vi "FastCalib.vi"(0 "Pixel to micron":dbl=1.58, 1 "No of each images":dbl, 2 "Template Path":path, 3 "coordinates":dbl[][](array[numeric]), 4 "Array 2":T2[](array[plugin-control])) -> (7 "angle in radian.":dbl, 8 "Mean":dbl[][](array[numeric]))   [LabVIEW 2016]
uses:
  <vilib>/vision/Measure.llb/Edge Options.ctl
  <vilib>/vision/Measure.llb/Edge Polarity.ctl
  <vilib>/Analysis/6fits.llb/Curve Fitting Criteria.ctl
  <vilib>/vision/NI_Vision_Development_Module.lvlib
  <resource>/objmgr/IMAQImage.rc
  <vilib>/Analysis/NI_AALBase.lvlib
  <vilib>/Analysis/NI_AALPro.lvlib
panel:
  in  "Tab Control":T1(tab)
  out "Y pixel":dbl
  out "X pixel":dbl
  out "angle.":dbl
  out "standard deviation":dbl[][](array[numeric])
  out "ratio of good position.":dbl[](array[numeric])
  in  "method":T3 items=["Least Square", "Least Absolute Residual", "Bisquare"]
  in  "Settings":T4={"Algorithm"=1, "Number of Matches Requested"=1, "Minimum Match Score"=800.0, "SubPixel Accuracy"=TRUE, "Rotation Angle Ranges"=[{"Start"=0.0, "End"=360.0}], "Show Search Area"=FALSE, "Show Result"=TRUE} {"Rotation Angle Ranges"."End" format="%.1f"; "Rotation Angle Ranges"."Start" format="%.1f"; "Minimum Match Score" min=0 max=1000 format="%.2f"; "Number of Matches Requested" min=1; "Algorithm" items=["All", "Low Discrepancy Sampling", "Grayscale Value Pyramid", "Gradients Pyramid"]}
  in  "Circle Fit Options":T5={"Process"=enum."Get First Edge", "Step Size"=3.0, "Max Pixel Radius"=3}
  in  "Options":T8={"Search  Direction"=1, "Edge Options"={"Edge Polarity"=0, "Kernel Size"=3, "Width"=3, "Minimum Edge Strength"=10.0, "Interpolation Type"=enum."Bilinear Fixed", "Data Processing Method"=enum."Average"}, "Show Search Area"=FALSE, "Show Search Lines"=FALSE, "Show Edges Found"=FALSE, "Show Result"=TRUE, "Search Area Color"=65280, "Search Lines Color"=255, "Edge Locations Color"=16776960, "Result Color"=16711680, "Overlay Group Name"=""} {"Search  Direction" items=["Outside to Inside", "Inside to Outside"]; "Edge Options"."Edge Polarity" items=["All Edges", "Rising Edges", "Falling Edges"]; "Edge Options"."Minimum Edge Strength" format="%.2f"; "Edge Options"."Width" step=2; "Edge Options"."Kernel Size" step=2}
  in  "Annulus ROI Descriptor":T9={"Global Rectangle"=[675, 567, 1751, 1642], "Contours"=[{"ID"=enum."External", "Type"=7, "Coordinates"=[1212, 1104, 85, 537, 0, 0]}]} {"Contours"."Type" items=["No Selection", "Point", "Line", "Rectangle", "Oval", "Polygon", "Freehand Region", "Annulus", "Unused2", "Unused3", "Broken Line", "Freehand Line", "Rotated Rectangle"]}
  out "Fitted Circle":T10 {"Average SNR (dB)" format="%.2f"; "Average Strength" format="%.2f"; "Roundness (Real-World)" format="%.2f"; "Radius (Real-World)" format="%.2f"; "Center (Real-World)"."Y" format="%.2f"; "Center (Real-World)"."X" format="%.2f"; "Radius (Pixels)" format="%.2f"; "Center (Pixels)"."Y" format="%.2f"; "Center (Pixels)"."X" format="%.2f"}
  out "Resulting ROI":T11
  out "Array":T2[](array[plugin-control])
  in  "No of pin":dbl=7.0
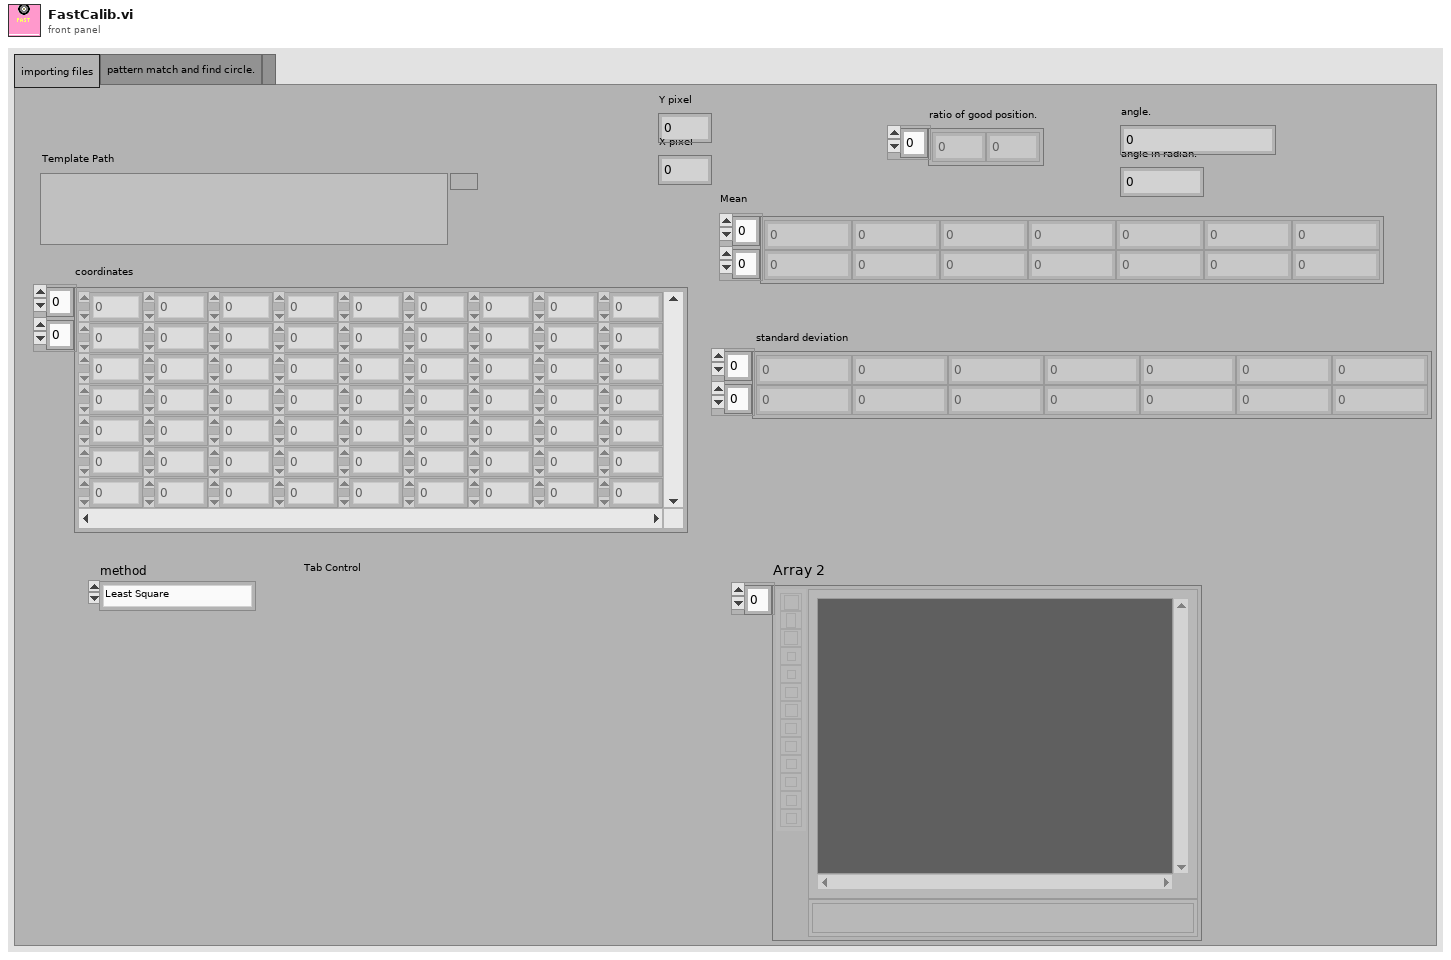
[diagram p1: front panel]
types:
  T1 = enum32{"importing files", "pattern match and find circle.", ""}
  T2 = typedef "IMAQ Image.ctl" = refnum<image>
  T3 = typedef "NI_AALPro.lvlib/Curve Fitting Criteria.ctl" = u16
  T4 = cluster{"Algorithm":i32, "Number of Matches Requested":i32, "Minimum Match Score":sgl, "SubPixel Accuracy":bool, "Rotation Angle Ranges":cluster{"Start":sgl, "End":sgl}[], "Show Search Area":bool, "Show Result":bool}
  T5 = cluster{"Process":enum16{"Get First Edge", "Get First + Last Edge", "Get All Edges", "Get Best Edge"}, "Step Size":dbl, "Max Pixel Radius":i32}
  T6 = typedef "Edge Options.ctl" = cluster{"Edge Polarity":T7, "Kernel Size":u32, "Width":u32, "Minimum Edge Strength":sgl, "Interpolation Type":enum32{"Zero Order", "Bilinear", "Quadratic", "Cubic", "Bilinear Fixed"}, "Data Processing Method":enum32{"Average", "Median"}}
  T7 = typedef "Edge Polarity.ctl" = u32
  T8 = cluster{"Search  Direction":u32, "Edge Options":T6, "Show Search Area":bool, "Show Search Lines":bool, "Show Edges Found":bool, "Show Result":bool, "Search Area Color":u32, "Search Lines Color":u32, "Edge Locations Color":u32, "Result Color":u32, "Overlay Group Name":string}
  T9 = cluster{"Global Rectangle":i32[], "Contours":cluster{"ID":enum32{"External", "Internal"}, "Type":u32, "Coordinates":i32[]}[]}
  T10 = cluster{"Center (Pixels)":cluster{"X":sgl, "Y":sgl}, "Radius (Pixels)":dbl, "Center (Real-World)":cluster{"X":sgl, "Y":sgl}, "Radius (Real-World)":dbl, "Roundness (Real-World)":dbl, "Average Strength":dbl, "Average SNR (dB)":dbl}
  T11 = cluster{sgl[], cluster{"ID":enum32{"External", "Internal"}, "Type":u32, "Coordinates":i32[]}[]}
  T12 = cluster{"ID":enum32{"External", "Internal"}, "Type":u32, "Coordinates":i32[]}[]
  T13 = cluster{"Position":cluster{"x":sgl, "y":sgl}, "Angle":sgl, "Scale":sgl, "Score":sgl, "Bounding Box":cluster{"x":sgl, "y":sgl}[]}[]
  T14 = cluster{"ID":enum32{"External", "Internal"}, "Type":u32, "Coordinates":i32[]}
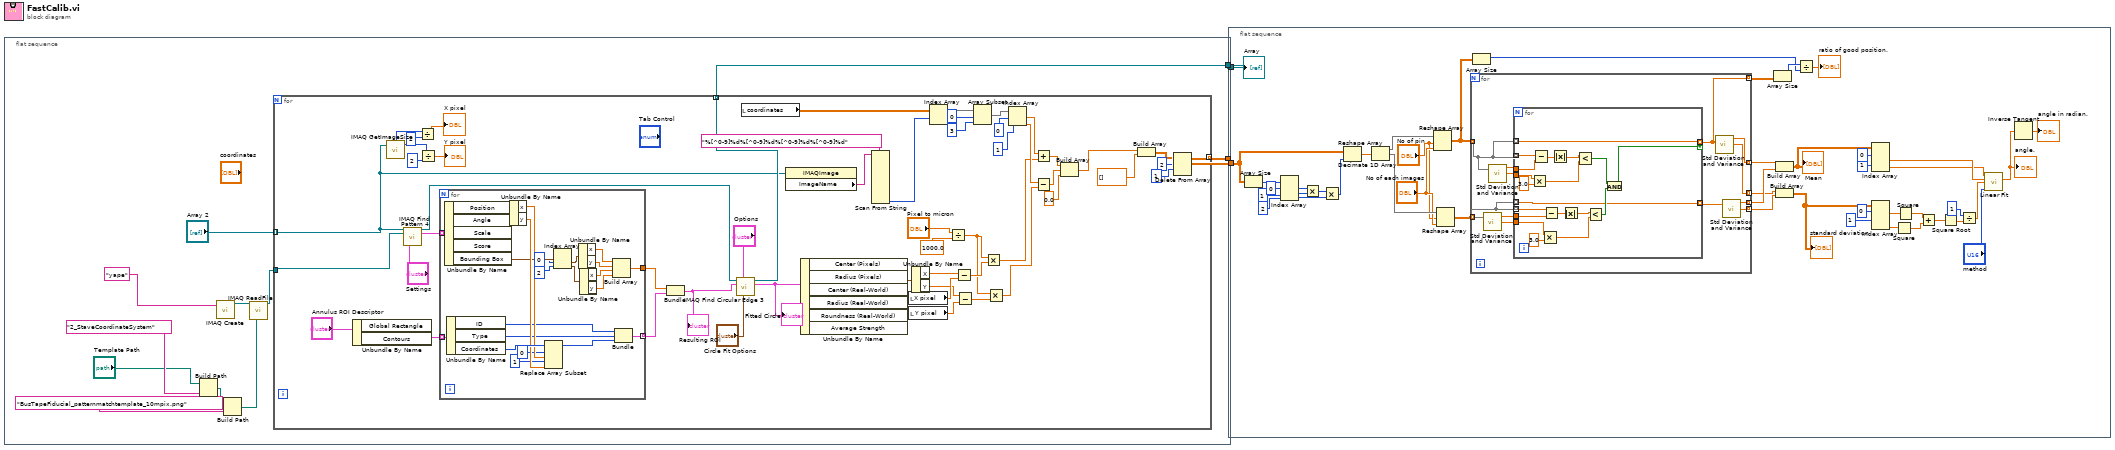
[diagram p0: block diagram]
diagram:
  n1 = flat-sequence {
    tunnel: [w10] -> w2
    tunnel: [w11] -> w1
    frame #0 {
      n2 = Build Path(base path="Template Path", name or relative path="2_StaveCoordinateSystem") -> (appended path=w6:path)
      n3 = call "IMAQ Create"("Image Name"="yape") -> ("New Image"=w13:T2)  [unwired: 4 in, 1 out]
      n4 = Build Path(base path=w6, name or relative path="BusTapeFiducial_patternmatchtemplate_10mpix.png") -> (appended path=w4:path)
      n5 = call "IMAQ ReadFile"("File Path"=w4, "Image"=w13) -> ("Image Out"=w12:T2)  [unwired: 5 in, 4 out]
      n6 = for {
        tunnel: w12 -> [w66]
        tunnel: [w40] -> w10 mode=indexing
        tunnel: [w29] -> w11 mode=indexing
        tunnel: "Array 2" -> [w14] mode=indexing
        n7 = Unbundle By Name("Annulus ROI Descriptor") -> ("Contours"=w62:T12)  [unwired: 1 out]
        n8 = call "IMAQ GetImageSize"("Image"=w14) -> ("Y Resolution"=w52:i32, "X Resolution"=w54:i32)  [unwired: 3 in, 1 out]
        n9 = call "IMAQ Find Pattern 4"("Image"=w14, "Template"=w66, "Settings"="Settings") -> ("Image Out"=w57:T2, "Matches (pixel)"=w64:T13)  [unwired: 6 in, 5 out]
        n10 = Divide(x=w54, y=2) -> (x/y=→"X pixel":dbl)
        n11 = Divide(x=w52, y=2) -> (x/y=→"Y pixel":dbl)
        n12 = for {
          tunnel: w64 -> [w88] mode=indexing
          tunnel: w62 -> [w86] mode=indexing
          tunnel: [w68] -> w61
          tunnel: [w67] -> w60 mode=indexing
          n13 = Unbundle By Name(w88) -> ("Position"=w87:cluster{"x":sgl, "y":sgl}, "Bounding Box"=w77:cluster{"x":sgl, "y":sgl}[])  [unwired: 3 out]
          n14 = Unbundle By Name(w86) -> ("ID"=w78:enum32{"External", "Internal"}, "Type"=w79:u32, "Coordinates"=w85:i32[])
          n15 = Unbundle By Name(w87) -> ("x"=w84:sgl, "y"=w83:sgl)
          n16 = Replace Array Subset(array=w85, new element #1=w84, index #1=0 ("index"), new element #2=w83, index #2=1 ("index")) -> (w80:i32[])
          n17 = Index Array(array=w77, index #1=0 ("index"), index #2=2 ("index")) -> (element #1=w73:cluster{"x":sgl, "y":sgl}, element #2=w74:cluster{"x":sgl, "y":sgl})
          n18 = Unbundle By Name(w73) -> ("x"=w69:sgl, "y"=w70:sgl)
          n19 = Unbundle By Name(w74) -> ("x"=w71:sgl, "y"=w72:sgl)
          n20 = Build Array(w69, w70, w71, w72) -> (w68:sgl[])
          n21 = Bundle("ID"=w78, "Type"=w79, "Coordinates"=w80) -> (w67:T14)  [unwired: 1 in]
        }
        n22 = Bundle(w61, w60) -> (w59:T11)  [unwired: 1 in]
        "Resulting ROI" <- w59
        n23 = call "IMAQ Find Circular Edge 3"("Circle Fit Options"="Circle Fit Options", "Options"="Options", "ROI Descriptor"=w59, "Image"=w57) -> ("Fitted Circle"=w56:T10, "Image Out"=w40:T2)  [unwired: 3 in, 3 out]
        "Fitted Circle" <- w56
        n24 = local read "coordinates"() -> (w42:dbl[][])
        n25 = property class="IMAQImage"(reference=w14) -> ("ImageName"=w44:string)  [unwired: 1 in, 2 out]
        n26 = Unbundle By Name(w56) -> ("Center (Pixels)"=w16:cluster{"X":sgl, "Y":sgl})  [unwired: 5 out]
        n27 = Scan From String(format string="%[^0-9]%d%[^0-9]%d%[^0-9]%d%[^0-9]%d", input string=w44) -> (output 8=w41:i32)  [unwired: 17 in, 3 out]
        n28 = local read "X pixel"() -> (w47:dbl)
        n29 = local read "Y pixel"() -> (w45:dbl)
        n30 = Unbundle By Name(w16) -> ("X"=w48:sgl, "Y"=w46:sgl)
        n31 = Index Array(array=w42, index (row)=w41) -> (element=w21:dbl[])  [unwired: 1 in]
        n32 = Divide(x="Pixel to micron", y=1000.0) -> (x/y=w33:dbl)
        n33 = Subtract(x=w48, y=w47) -> (x-y=w34:dbl)
        n34 = Subtract(x=w46, y=w45) -> (x-y=w35:dbl)
        n35 = Array Subset(array=w21, index=0, length=3) -> (w15:dbl[])
        n36 = Multiply(x=w33, y=w34) -> (x*y=w20:dbl)
        n37 = Multiply(x=w33, y=w35) -> (x*y=w19:dbl)
        n38 = Index Array(array=w15, index #1=0 ("index"), index #2=1 ("index")) -> (element #1=w24:dbl, element #2=w25:dbl)
        n39 = Add(x=w24, y=w20) -> (x+y=w28:dbl)
        n40 = Subtract(x=w25, y=w19) -> (x-y=w27:dbl)
        n41 = Build Array(w28, w27, 0.0 ("element")) -> (w26:dbl[])
        n42 = Build Array(w26, dbl[] [] ("element")) -> (w18:dbl[][])
        n43 = Delete From Array(array=w18, length=2, index (row)=1) -> (array with subset deleted=w29:dbl[][])  [unwired: 1 in, 1 out]
      }
    }
  }
  n44 = flat-sequence {
    tunnel: w2 -> [w133]
    tunnel: w1 -> [w124]
    frame #0 {
      n45 = Array Size(array=w124) -> (size(s)=w132:i32[])
      n46 = Index Array(array=w132, index #1=0 ("index"), index #2=1 ("index"), index #3=2 ("index")) -> (element #1=w128:i32, element #2=w127:i32, element #3=w125:i32)
      n47 = Multiply(x=w128, y=w127) -> (x*y=w126:i32)
      n48 = Multiply(x=w126, y=w125) -> (x*y=w123:i32)
      n49 = Reshape Array(w124, w123) -> (w122:dbl[])
      n50 = Decimate 1D Array(w122) -> (w121:dbl[], w120:dbl[])  [unwired: 1 out]
      n51 = Reshape Array(w121, "No of pin", "No of each images") -> (w114:dbl[][])
      n52 = Reshape Array(w120, "No of pin", "No of each images") -> (w115:dbl[][])
      n53 = for {
        tunnel: w115 -> [w134] mode=indexing
        tunnel: [w140] -> w99 mode=indexing
        tunnel: [w139] -> w117 mode=indexing
        tunnel: w114 -> [w135] mode=indexing
        tunnel: [w138] -> w89 mode=indexing
        tunnel: [w137] -> w113 mode=indexing
        tunnel: [w136] -> w90 mode=indexing
        n54 = call <vilib>:"Std Deviation and Variance.vi"("X"=w134) -> ("mean"=w143:dbl, "standard deviation"=w142:dbl)  [unwired: 1 in, 1 out]
        n55 = call <vilib>:"Std Deviation and Variance.vi"("X"=w135) -> ("mean"=w144:dbl, "standard deviation"=w145:dbl)  [unwired: 1 in, 1 out]
        n56 = for {
          tunnel: w135 -> [w150] mode=indexing
          tunnel: [w147] -> w139 mode=indexing if=w164
          tunnel: w145 -> [w163]
          tunnel: w144 -> [w161]
          tunnel: w134 -> [w149] mode=indexing
          tunnel: w143 -> [w153]
          tunnel: w142 -> [w152]
          tunnel: [w146] -> w141 mode=indexing
          tunnel: w135 -> [w147] mode=indexing
          tunnel: w134 -> [w146] mode=indexing
          n57 = Multiply(x=w163, y=3.0 ("x")) -> (x*y=w158:dbl)
          n58 = Subtract(x=w150, y=w161) -> (x-y=w160:dbl)
          n59 = Multiply(x=w152, y=3.0 ("x")) -> (x*y=w154:dbl)
          n60 = Subtract(x=w149, y=w153) -> (x-y=w156:dbl)
          n61 = Absolute Value(x=w160) -> (abs(x)=w159:dbl)
          n62 = Absolute Value(x=w156) -> (abs(x)=w155:dbl)
          n63 = Less?(x=w159, y=w158) -> (x < y?=w157:bool)
          n64 = Less?(x=w155, y=w154) -> (x < y?=w151:bool)
          n65 = And(x=w157, y=w151) -> (x .and. y?=w164:bool)
        }
        n66 = call <vilib>:"Std Deviation and Variance.vi"("X"=w139) -> ("mean"=w140:dbl, "standard deviation"=w138:dbl)  [unwired: 1 in, 1 out]
        n67 = call <vilib>:"Std Deviation and Variance.vi"("X"=w141) -> ("mean"=w136:dbl, "standard deviation"=w137:dbl)  [unwired: 1 in, 1 out]
      }
      n68 = Array Size(array=w114) -> (size(s)=w112:i32[])
      n69 = Array Size(array=w117) -> (size(s)=w116:i32[])
      n70 = Build Array(w99, w90) -> (w96:dbl[][])
      "Mean" <- w96
      n71 = Build Array(w89, w113) -> (w110:dbl[][])
      "standard deviation" <- w110
      n72 = Divide(x=w116, y=w112) -> (x/y=→"ratio of good position.":dbl[])
      n73 = Index Array(array=w96, index (row) #1=0 ("index (row)"), index (row) #2=1 ("index (row)")) -> (element #1=w93:dbl[], element #2=w92:dbl[])  [unwired: 2 in]
      n74 = Index Array(array=w110, index (row) #1=0 ("index (row)"), index (row) #2=1 ("index (row)")) -> (element #1=w106:dbl[], element #2=w107:dbl[])  [unwired: 2 in]
      n75 = Square(x=w107) -> (x^2=w105:dbl[])
      n76 = Square(x=w106) -> (x^2=w104:dbl[])
      n77 = Add(x=w104, y=w105) -> (x+y=w103:dbl[])
      n78 = Square Root(x=w103) -> (sqrt(x)=w102:dbl[])
      n79 = Divide(x=1, y=w102) -> (x/y=w100:dbl[])
      n80 = call <vilib>:"Linear Fit.vi"("Y"=w92, "X"=w93, "Weight"=w100, "method"="method") -> ("slope"=w98:dbl)  [unwired: 7 in, 4 out]
      "angle." <- w98
      n81 = Inverse Tangent(1:w98) -> (0:→"angle in radian.":dbl)
      "Array" <- w133
    }
  }
